vi "Lockin-4461 IV mode trigger and wait.vi"(8 "error in (no error)":errorcluster) -> (0 "error out":errorcluster)   [LabVIEW 2013]
panel:
  in  "Channels: AO":T1={"AO amp (V)"=[1.0, 0.0, 0.0, 0.0, 0.0, 0.0, 0.0, 0.0], "AO DC (V)"=[0.0, 0.0, 0.0, 0.0, 0.0, 0.0, 0.0, 0.0], "AO f (Hz)"=[1.0, 1.0, 1.0, 1.0, 1.0, 1.0, 1.0, 1.0], "AO phi (deg)"=[0.0, 0.0, 0.0, 0.0, 0.0, 0.0, 0.0, 0.0], "function"=[enum."Triangle Wave", enum."Sine Wave", enum."Sine Wave", enum."Sine Wave", enum."Sine Wave", enum."Sine Wave", enum."Sine Wave", enum."Sine Wave"]} {"AO DC (V)" format="%#_6p"; "AO amp (V)" format="%#_6p"}
  in  "y":bool
  out "timer (s)":dbl=1.2239999771118164
  # "This VI triggers the lockin and waits until the acquisition is complete"
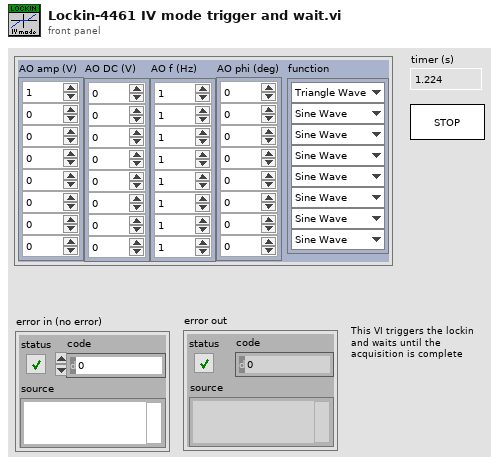
[diagram p1: front panel]
types:
  T1 = cluster{"AO amp (V)":dbl[], "AO DC (V)":dbl[], "AO f (Hz)":dbl[], "AO phi (deg)":dbl[], "function":enum16{"Sine Wave", "Triangle Wave", "Square Wave", "Sawtooth Wave"}[]}
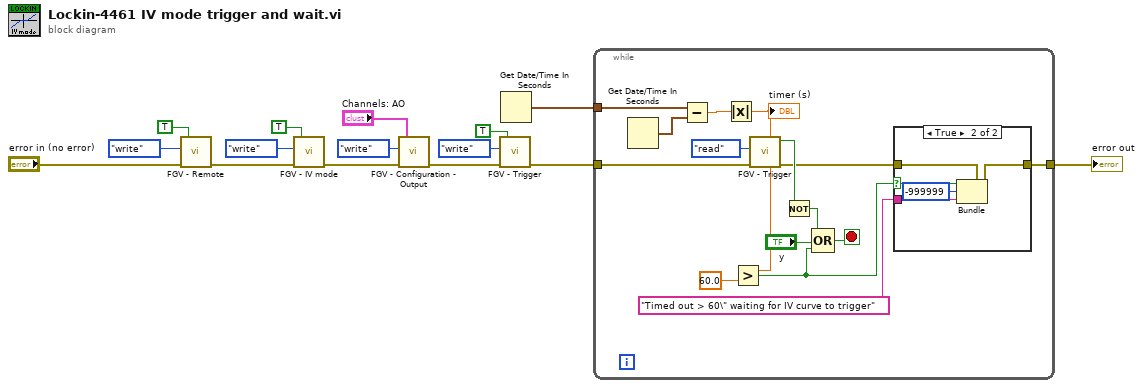
[diagram p0: block diagram]
diagram:
  n1 = call "FGV - Remote.vi"("error in"="error in (no error)", "Function"=enum16{"write", "read"}."write", "Remote Mode"=TRUE ("Trigger")) -> ("error out"=w7:errorcluster)  [unwired: 3 in, 1 out]
  n2 = call "FGV - IV mode.vi"("error in"=w7, "Function"=enum16{"write", "read"}."write", "IV mode"=TRUE ("Trigger")) -> ("error out"=w4:errorcluster)  [unwired: 3 in, 1 out]
  n3 = call "FGV - Configuration - Output.vi"("error in"=w4, "Function"=enum16{"write", "read"}."write", "Channels: AO"="Channels: AO") -> ("error out"=w3:errorcluster)  [unwired: 3 in, 1 out]
  n4 = call "FGV - Trigger.vi"("error in"=w3, "Function"=enum16{"write", "read"}."write", "Trigger"=TRUE) -> ("error out"=w13:errorcluster)  [unwired: 3 in, 1 out]
  n5 = Get Date/Time In Seconds() -> (seconds since 1Jan1904=w12:timestamp)
  n6 = while {
    tunnel: w13 -> [w25]
    tunnel: w12 -> [w28]
    tunnel: [w16] -> w11
    stop <- w24 stop-if-true
    n7 = Get Date/Time In Seconds() -> (seconds since 1Jan1904=w27:timestamp)
    n8 = Subtract(x=w28, y=w27) -> (x-y=w26:dbl)
    n9 = Absolute Value(x=w26) -> (abs(x)=w21:dbl)
    "timer (s)" <- w21
    n10 = Greater?(x=w21, y=60.0) -> (0:w18:bool)
    n11 = call "FGV - Trigger.vi"("error in"=w25, "Function"=enum16{"write", "read"}."read") -> ("error out"=w17:errorcluster, "Trigger 2"=w29:bool)  [unwired: 4 in]
    n12 = Not(x=w29) -> (.not. x?=w23:bool)
    n13 = Compound Arithmetic op=OR(w23, "y", w18) -> (w24:bool)
    n14 = case shown="True" w18 {
      selector: w18 -> [_ w34]
      tunnel: "Timed out > 60\" waiting for IV curve to trigger" ("source") -> [_ w36]
      tunnel: w17 -> [w31 w35]
      tunnel: [w31 w33] -> w16
      frame False {
      }
      frame True {
        n15 = Bundle(cluster=w35, "status"=w34, "code"=-999999, "source"=w36) -> (w33:errorcluster)
      }
    }
  }
  "error out" <- w11
